vi "S2C_OM8257_Poly_TestBed.vi"() -> ()   [LabVIEW 2015]
uses:
  S2C_OM8257_Poly_Initialize.vi
  S2C_OM8257_Poly_ACW.vi
  S2C_OM8257_Poly_LLT.vi
  S2C_OM8257_Poly_GND.vi
  S2C_OM8257_Poly_RUN.vi
  S2C_OM8257_Poly_Prompt.vi
  S2C_OM8257_Poly_Execute.vi
  S2C_OM8257_Poly_NewFile.vi
  S2C_OM8257_Poly_LoadFile.vi
  S2C_OM8257_Poly_DeleteFile.vi
  S2C_OM8257_Poly_QueryFilename.vi
  S2C_OM8257_Poly_FileStopFail.vi
  S2C_OM8257_Poly_QueryStepSelect.vi
  S2C_OM8257_Poly_ReadResult.vi
  S2C_OM8257_Poly_ReadTestDisplay.vi
  S2C_OM8257_Poly_SwReboot.vi
panel:
  out "Error Out":errorcluster
  in  "Error In":errorcluster
  out "Response":T1
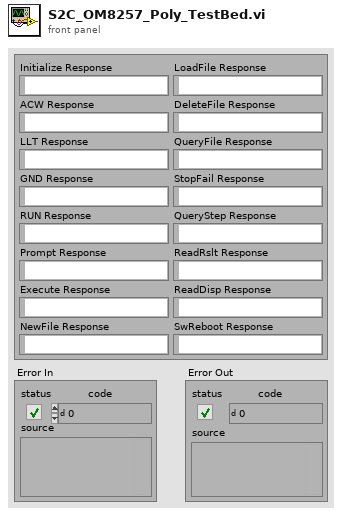
[diagram p1: front panel]
types:
  T1 = cluster{"Initialize Response":string, "ACW Response":string, "LLT Response":string, "GND Response":string, "RUN Response":string, "Prompt Response":string, "Execute Response":string, "NewFile Response":string, "LoadFile Response":string, "DeleteFile Response":string, "QueryFile Response":string, "StopFail Response":string, "QueryStep Response":string, "ReadRslt Response":string, "ReadDisp Response":string, "SwReboot Response":string}
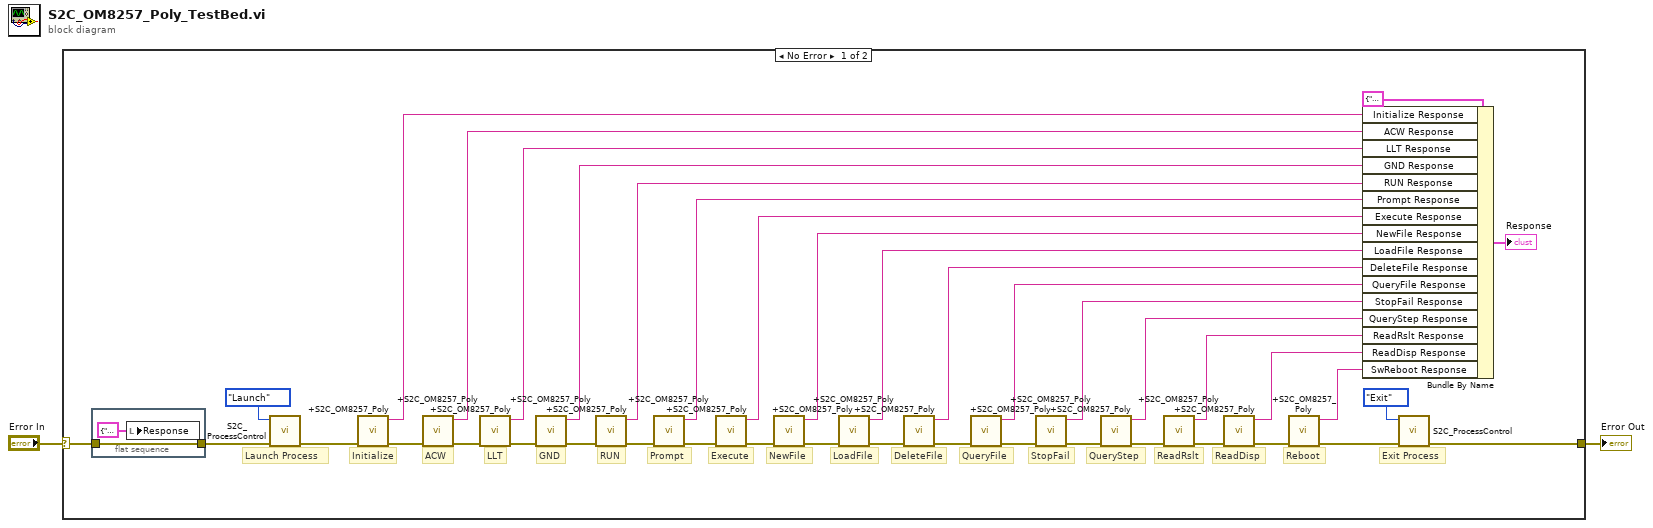
[diagram p0: block diagram]
diagram:
  n1 = case shown="No Error" "Error In" {
    selector: "Error In" -> [w37 w45]
    tunnel: [w39 w45] -> w1
    frame No Error {
      # "Reboot"
      # "ReadDisp"
      # "ReadRslt"
      # "QueryStep"
      # "StopFail"
      # "QueryFile"
      # "DeleteFile"
      # "LoadFile"
      # "NewFile"
      # "Execute"
      # "Prompt"
      # "RUN"
      # "GND"
      # "LLT"
      # "ACW"
      # "Exit Process"
      # "Initialize"
      # "Launch Process"
      n2 = flat-sequence {
        tunnel: w37 -> [w44]
        tunnel: [w44] -> w36
        frame #0 {
          n3 = local write "Response"(T1 {"Initialize Response"="", "ACW Response"="", "LLT Response"="", "GND Response"="", "RUN Response"="", "Prompt Response"="", "Execute Response"="", "NewFile Response"="", "LoadFile Response"="", "DeleteFile Response"="", "QueryFile Response"="", "StopFail Response"="", "QueryStep Response"="", "ReadRslt Response"="", "ReadDisp Response"="", "SwReboot Response"=""} ("Response")) -> ()
        }
      }
      n4 = call "S2C_ProcessControl.vi"("Error In"=w36, "Action"=enum16{"Launch", "Exit"}."Launch") -> ("Error Out"=w41:errorcluster)  [unwired: 9 in]
      n5 = call-poly "+S2C_OM8257_Poly.vi"("Error In"=w41) -> ("Error Out"=w35:errorcluster, "Response"=w38:string)  [unwired: 9 in]
      n6 = call-poly "+S2C_OM8257_Poly.vi"("Error In"=w35) -> ("Error Out"=w34:errorcluster, "Response"=w18:string)  [unwired: 9 in]
      n7 = call-poly "+S2C_OM8257_Poly.vi"("Error In"=w34) -> ("Error Out"=w33:errorcluster, "Response"=w17:string)  [unwired: 9 in]
      n8 = call-poly "+S2C_OM8257_Poly.vi"("Error In"=w33) -> ("Error Out"=w32:errorcluster, "Response"=w16:string)  [unwired: 9 in]
      n9 = call-poly "+S2C_OM8257_Poly.vi"("Error In"=w32) -> ("Error Out"=w31:errorcluster, "Response"=w15:string)  [unwired: 9 in]
      n10 = call-poly "+S2C_OM8257_Poly.vi"("Error In"=w31) -> ("Error Out"=w30:errorcluster, "Response"=w14:string)  [unwired: 9 in]
      n11 = call-poly "+S2C_OM8257_Poly.vi"("Error In"=w30) -> ("Error Out"=w29:errorcluster, "Response"=w13:string)  [unwired: 9 in]
      n12 = call-poly "+S2C_OM8257_Poly.vi"("Error In"=w29) -> ("Error Out"=w28:errorcluster, "Response"=w12:string)  [unwired: 9 in]
      n13 = call-poly "+S2C_OM8257_Poly.vi"("Error In"=w28) -> ("Error Out"=w27:errorcluster, "Response"=w11:string)  [unwired: 9 in]
      n14 = call-poly "+S2C_OM8257_Poly.vi"("Error In"=w27) -> ("Error Out"=w26:errorcluster, "Response"=w10:string)  [unwired: 9 in]
      n15 = call-poly "+S2C_OM8257_Poly.vi"("Error In"=w26) -> ("Error Out"=w25:errorcluster, "Response"=w9:string)  [unwired: 9 in]
      n16 = call-poly "+S2C_OM8257_Poly.vi"("Error In"=w25) -> ("Error Out"=w24:errorcluster, "Response"=w8:string)  [unwired: 9 in]
      n17 = call-poly "+S2C_OM8257_Poly.vi"("Error In"=w24) -> ("Error Out"=w22:errorcluster, "Response"=w7:string)  [unwired: 9 in]
      n18 = call-poly "+S2C_OM8257_Poly.vi"("Error In"=w22) -> ("Error Out"=w23:errorcluster, "Response"=w6:string)  [unwired: 9 in]
      n19 = call-poly "+S2C_OM8257_Poly.vi"("Error In"=w23) -> ("Error Out"=w21:errorcluster, "Response"=w5:string)  [unwired: 9 in]
      n20 = call-poly "+S2C_OM8257_Poly.vi"("Error In"=w21) -> ("Error Out"=w3:errorcluster, "Response"=w4:string)  [unwired: 9 in]
      n21 = Bundle By Name(cluster=T1 {"Initialize Response"="", "ACW Response"="", "LLT Response"="", "GND Response"="", "RUN Response"="", "Prompt Response"="", "Execute Response"="", "NewFile Response"="", "LoadFile Response"="", "DeleteFile Response"="", "QueryFile Response"="", "StopFail Response"="", "QueryStep Response"="", "ReadRslt Response"="", "ReadDisp Response"="", "SwReboot Response"=""} ("Response"), "Initialize Response"=w38, "ACW Response"=w18, "LLT Response"=w17, "GND Response"=w16, "RUN Response"=w15, "Prompt Response"=w14, "Execute Response"=w13, "NewFile Response"=w12, "LoadFile Response"=w11, "DeleteFile Response"=w10, "QueryFile Response"=w9, "StopFail Response"=w8, "QueryStep Response"=w7, "ReadRslt Response"=w6, "ReadDisp Response"=w5, "SwReboot Response"=w4) -> (→"Response":T1)
      n22 = call "S2C_ProcessControl.vi"("Error In"=w3, "Action"=enum16{"Launch", "Exit"}."Exit") -> ("Error Out"=w39:errorcluster)  [unwired: 9 in]
    }
    frame Error {
    }
  }
  "Error Out" <- w1
